vi "day 10 Main.vi"() -> ()   [LabVIEW 2020]
uses:
  eddc149c-0d1a-4f58-a217-c9a07680dd4e.vi
  <vilib>/Comparison/Equal/Equal Functor/Equal Functor.lvclass
  state --enum.ctl
panel:
  out "CRT":bool[][](array[boolean])
  out "sum":i32
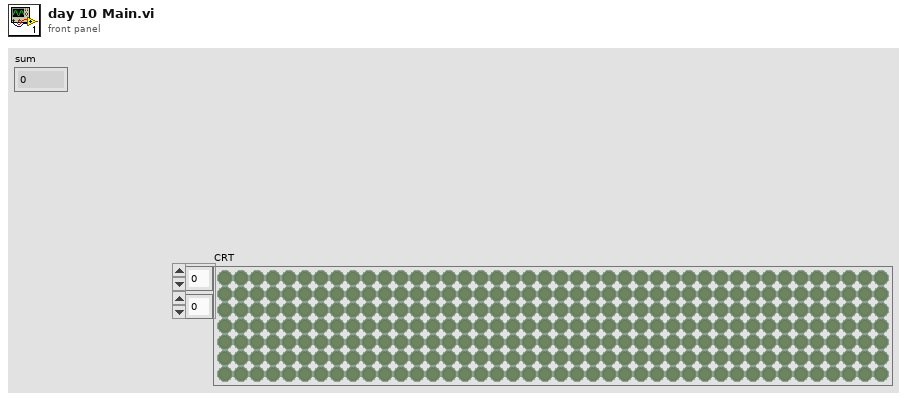
[diagram p1: front panel]
types:
  T1 = typedef "state --enum.ctl" = enum16{"Idle", "Executing"}
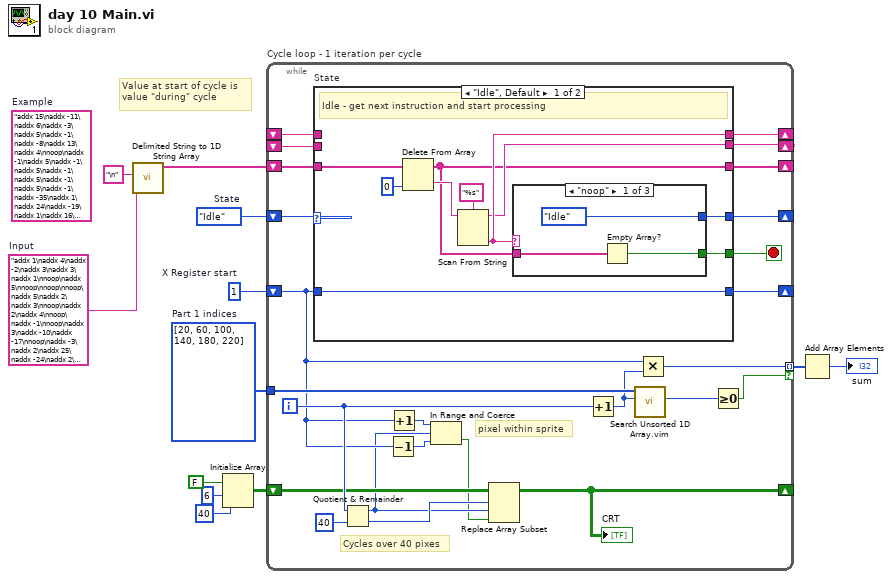
[diagram p0: block diagram]
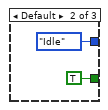
[diagram p2: hidden frame]
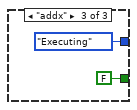
[diagram p3: hidden frame]
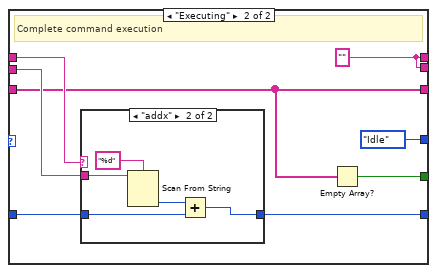
[diagram p4: hidden frame]
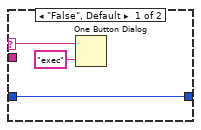
[diagram p5: hidden frame]
diagram:
  w12 = state_--enum."Idle"  # State
  w5 = "addx 1\naddx 4\naddx -2\naddx 3\naddx 3\naddx 1\nnoop\naddx 5\nnoop\nnoop\nnoop\naddx 5\naddx 2\naddx 3\nnoop\naddx 2\naddx 4\nnoop\naddx -1\nnoop\naddx 3\naddx -10\naddx -17\nnoop\naddx -3\naddx 2\naddx 25\naddx -24\naddx 2\naddx 5\naddx 2\naddx 3\nnoop\naddx 2\naddx 14\naddx -9\nnoop\naddx 5\nnoop\nnoop\naddx -2\naddx 5\naddx 2\naddx -5\nnoop\nnoop\naddx -19\naddx -11\naddx 5\naddx 3\nnoop\naddx 2\naddx 3\naddx -2\naddx 2\nnoop\naddx 3\naddx 4\nnoop\nnoop\naddx 5\nnoop\nnoop\nnoop\naddx 5\naddx -3\naddx 8\nnoop\naddx -15\nnoop\naddx -12\naddx -9\nnoop\naddx 6\naddx 7\naddx -6\naddx 4\nnoop\nnoop\nnoop\naddx 4\naddx 1\naddx 5\naddx -11\naddx 29\naddx -15\nnoop\naddx -12\naddx 17\naddx 7\nnoop\nnoop\naddx -32\naddx 3\naddx -8\naddx 7\nnoop\naddx -2\naddx 5\naddx 2\naddx 6\naddx -8\naddx 5\naddx 2\naddx 5\naddx 17\naddx -12\naddx -2\nnoop\nnoop\naddx 7\naddx 9\naddx -8\naddx 2\naddx -33\naddx -1\naddx 2\nnoop\naddx 26\naddx -22\naddx 19\naddx -16\naddx 8\naddx -1\naddx 3\naddx -2\naddx 2\naddx -17\naddx 24\naddx 1\nnoop\naddx 5\naddx -1\nnoop\naddx 5\nnoop\nnoop\naddx 1\nnoop\nnoop"  # Input
  w8 = i32[] [20, 60, 100, 140, 180, 220]  # Part 1 indices
  (unwired) "addx 15\naddx -11\naddx 6\naddx -3\naddx 5\naddx -1\naddx -8\naddx 13\naddx 4\nnoop\naddx -1\naddx 5\naddx -1\naddx 5\naddx -1\naddx 5\naddx -1\naddx 5\naddx -1\naddx -35\naddx 1\naddx 24\naddx -19\naddx 1\naddx 16\naddx -11\nnoop\nnoop\naddx 21\naddx -15\nnoop\nnoop\naddx -3\naddx 9\naddx 1\naddx -3\naddx 8\naddx 1\naddx 5\nnoop\nnoop\nnoop\nnoop\nnoop\naddx -36\nnoop\naddx 1\naddx 7\nnoop\nnoop\nnoop\naddx 2\naddx 6\nnoop\nnoop\nnoop\nnoop\nnoop\naddx 1\nnoop\nnoop\naddx 7\naddx 1\nnoop\naddx -13\naddx 13\naddx 7\nnoop\naddx 1\naddx -33\nnoop\nnoop\nnoop\naddx 2\nnoop\nnoop\nnoop\naddx 8\nnoop\naddx -1\naddx 2\naddx 1\nnoop\naddx 17\naddx -9\naddx 1\naddx 1\naddx -3\naddx 11\nnoop\nnoop\naddx 1\nnoop\naddx 1\nnoop\nnoop\naddx -13\naddx -19\naddx 1\naddx 3\naddx 26\naddx -30\naddx 12\naddx -1\naddx 3\naddx 1\nnoop\nnoop\nnoop\naddx -9\naddx 18\naddx 1\naddx 2\nnoop\nnoop\naddx 9\nnoop\nnoop\nnoop\naddx -1\naddx 2\naddx -37\naddx 1\naddx 3\nnoop\naddx 15\naddx -21\naddx 22\naddx -6\naddx 1\nnoop\naddx 2\naddx 1\nnoop\naddx -10\nnoop\nnoop\naddx 20\naddx 1\naddx 2\naddx 2\naddx -6\naddx -11\nnoop\nnoop\nnoop"  # Example
  w11 = 1  # X Register start
  # "Value at start of cycle is value \"during\" cycle"
  n1 = call <vilib>:"Delimited String to 1D String Array.vi"("delimiter"="\n", "delimited string"=w5) -> ("string array"=w9:string[])  [unwired: 9 in]
  n2 = Initialize Array(FALSE, 6 ("dimension size"), 40 ("dimension size")) -> (w1:bool[][])
  n3 = while "Cycle loop - 1 iteration per cycle" {
    shift-right: [w35] -> _
    shift-left: w12 -> [w37]
    shift-right: [w30] -> _
    shift-left: w9 -> [w36]
    shift-right: [w24] -> _
    shift-left: w11 -> [w18]
    shift-right: [w34] -> _
    shift-left: _ -> [w33]
    shift-right: [w32] -> _
    shift-left: _ -> [w31]
    tunnel: w8 -> [w28]
    tunnel: [w26] -> w7 mode=indexing if=w23
    shift-right: [w13] -> _
    shift-left: w1 -> [w20]
    i -> [w22]
    stop <- w29 stop-if-true
    # "pixel within sprite"
    # "Cycles over 40 pixes"
    n4 = case "State" shown="\"Idle\", Default" w37 {
      tunnel: w36 -> [w40 w56]
      tunnel: [w39 w56] -> w30
      tunnel: [w45 state_--enum."Idle" ("State 2")] -> w35
      tunnel: w18 -> [w44 w58]
      tunnel: [w44 w57] -> w24
      tunnel: [w42 w61] -> w34
      tunnel: w33 -> [_ w60]
      tunnel: [w41 w61] -> w32
      tunnel: w31 -> [_ w59]
      tunnel: [w38 w55] -> w29
      frame "Idle", Default {
        # "Idle - get next instruction and start processing"
        n5 = Delete From Array(array=w40, index=0) -> (deleted portion=w43:string, array with subset deleted=w39:string[])  [unwired: 1 in]
        n6 = Scan From String(format string="%s", input string=w43) -> (remaining string=w41:string, output 1=w42:string)  [unwired: 3 in, 2 out]
        n7 = case shown="\"noop\"" w42 {
          tunnel: [state_--enum."Idle" ("State 2") state_--enum."Idle" ("State 2") state_--enum."Executing" ("State 2")] -> w45
          tunnel: w39 -> [w49 _ _]
          tunnel: [w48 TRUE ("empty?") FALSE ("empty?")] -> w38
          frame "noop" {
            n8 = Empty Array?(array=w49) -> (empty?=w48:bool)
          }
          frame Default {
          }
          frame "addx" {
          }
        }
      }
      frame "Executing" {
        w61 = ""
        # "Complete command execution"
        n9 = case shown="\"addx\"" w60 {
          selector: w60 -> [w64 _]
          tunnel: w59 -> [_ w70]
          tunnel: w58 -> [w65 w67]
          tunnel: [w65 w66] -> w57
          frame "False", Default {
            n10 = One Button Dialog(message=w64, button name ("OK")="exec") -> ()  [unwired: 1 out]
          }
          frame "addx" {
            n11 = Scan From String(format string="%d", input string=w70) -> (output 1=w68:i32)  [unwired: 3 in, 3 out]
            n12 = Add(x=w68, y=w67) -> (x+y=w66:i32)
          }
        }
        n13 = Empty Array?(array=w56) -> (empty?=w55:bool)
      }
    }
    n14 = Quotient & Remainder(x=w22, y=40) -> (x-y*floor(x/y)=w15:i32, floor(x/y)=w19:i32)
    n15 = Decrement(x=w18) -> (x-1=w16:i32)
    n16 = Increment(x=w18) -> (x+1=w17:i32)
    n17 = In Range and Coerce(upper limit=w17, x=w15, lower limit=w16) -> (In Range?=w14:bool)  [unwired: 1 out]
    n18 = Replace Array Subset(array=w20, new element=w14, index (row)=w19, index (col)=w15) -> (w13:bool[][])
    "CRT" <- w13
    n19 = Increment(x=w22) -> (x+1=w25:i32)
    n20 = call "Search Unsorted 1D Array.vim"("element"=w25, "unsorted 1D array"=w28) -> ("index of element"=w27:i32)  [unwired: 9 in]
    n21 = Multiply(x=w18, y=w25) -> (x*y=w26:i32)
    n22 = Greater Or Equal To 0?(x=w27) -> (x >= 0?=w23:bool)
  }
  n23 = Add Array Elements(numeric array=w7) -> (sum=→"sum":i32)
